vi "Actor Core.vi"(8 "error in":errorcluster, 11 "Panel Actor in":refnum<class "Panel Actor.lvclass">) -> (0 "error out":errorcluster, 3 "Actor out":refnum<class "Actor.lvclass">)   [LabVIEW 2023, in "Panel Actor.lvlib" / "Panel Actor.lvclass"]
doc: "The user interface for this panel.\n\n----\nPlease see the following web address for additional documentation and tutorial information:\nhttp://www.mooregoodideas.com/mgi-panel-manager/\n\nAuthor: Derek Trepanier\n\nCopyright (c) 2018, Moore Good Ideas, Inc.\n\nAll rights reserved.\n\nRedistribution and use in source and binary forms, with or without modification, are permitted provided that the following conditions are met:\n\n * Redistributions of source code must retain the above copyright notice, this list of conditions and the following disclaimer.\n * Redistributions in binary form must reproduce the above copyright notice, this list of conditions and the following disclaimer in the documentation and/or other materials provided with the distribution.\n * Neither the name of Moore Good Ideas, Inc. nor the names of its contributors may be used to endorse or promote products derived from this software without specific prior written permission.\n\nTHIS SOFTWARE IS PROVIDED BY THE COPYRIGHT HOLDERS AND CONTRIBUTORS \"AS IS\" AND ANY EXPRESS OR IMPLIED WARRANTIES, INCLUDING, BUT NOT LIMITED TO, THE IMPLIED WARRANTIES OF MERCHANTABILITY AND FITNESS FOR A PARTICULAR PURPOSE ARE DISCLAIMED. IN NO EVENT SHALL THE COPYRIGHT OWNER OR CONTRIBUTORS BE LIABLE FOR ANY DIRECT, INDIRECT, INCIDENTAL, SPECIAL, EXEMPLARY, OR CONSEQUENTIAL DAMAGES (INCLUDING, BUT NOT LIMITED TO, PROCUREMENT OF SUBSTITUTE GOODS OR SERVICES; LOSS OF USE, DATA, OR PROFITS; OR BUSINESS INTERRUPTION) HOWEVER CAUSED AND ON ANY THEORY OF LIABILITY, WHETHER IN CONTRACT, STRICT LIABILITY, OR TORT (INCLUDING NEGLIGENCE OR OTHERWISE) ARISING IN ANY WAY OUT OF THE USE OF THIS SOFTWARE, EVEN IF ADVISED OF THE POSSIBILITY OF SUCH DAMAGE."
uses:
  Library/Panel Actor.lvclass
  Panel/Panel/Panel.lvclass
  builds/Framework/Monitored Actor.lvlibp/Actor Monitor/Actor Monitor/Actor Monitor.lvclass
  builds/Framework/Actor Framework.lvlibp/1abvi3w/vi.lib/ActorFramework/Actor/Actor.lvclass
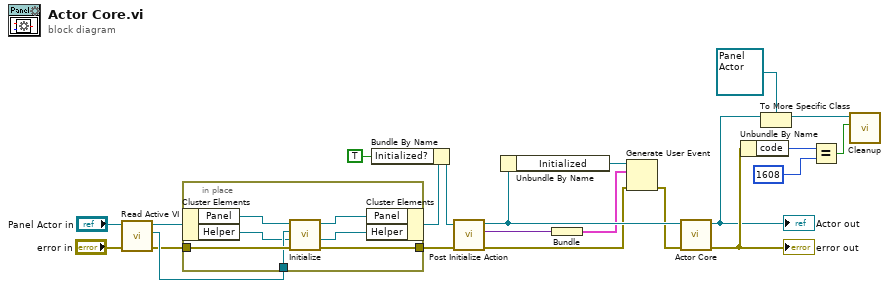
[diagram p0: block diagram]
diagram:
  n1 = call "Read Active VI.vi"("error in (no error)"="error in", "Panel Actor in"="Panel Actor in") -> ("error out"=w12:errorcluster, "Active VI ref"=w14:refnum<vi>, "Panel Actor out"=w15:refnum<class "Panel Actor.lvclass">)  [unwired: 7 in]
  n2 = in-place {
    in-place-border: w12 -> [w29]
    in-place-border: w14 -> [w27]
    in-place-border: [w26] -> w22
    n3 = in-place-cluster #1(w15) -> ("Panel"=w28:refnum<class "Panel.lvclass">, "Helper"=w23:refnum<class "Panel Helper.lvclass">)
    n4 = call "Initialize.vi"("error in (no error)"=w29, "My Helper in"=w23, "VI Refnum"=w27, "Panel In"=w28) -> ("error out"=w26:errorcluster, "My Helper out"=w24:refnum<class "Panel Helper.lvclass">, "Panel Out"=w25:refnum<class "Panel.lvclass">)  [unwired: 5 in]
    n5 = in-place-cluster #1("Panel"=w25, "Helper"=w24) -> (w20:refnum<class "Panel Actor.lvclass">)
  }
  n6 = Bundle By Name(cluster=w20, "Initialized?"=TRUE) -> (w8:refnum<class "Panel Actor.lvclass">)
  n7 = call-dynamic "Post Initialize Action.vi"("error in (no error)"=w22, "Panel Actor in"=w8) -> ("error out"=w4:errorcluster, "Init Event Data"=w2:variant, "Panel Actor out"=w6:refnum<class "Panel Actor.lvclass">)  [unwired: 7 in]
  n8 = Unbundle By Name(w6) -> ("Initialized"=w5:refnum<user-event>)
  n9 = Bundle("Init Event Data"=w2) -> (w1:cluster{"Init Event Data":variant})  [unwired: 1 in]
  n10 = Generate User Event(user event=w5, event data cluster=w1, error in=w4) -> (error out=w3:errorcluster)  [unwired: 1 in, 1 out]
  n11 = call-parent "Actor Core.vi"("error in"=w3, "Actor in"=w6) -> ("error out"=w19:errorcluster, "Actor out"=w10:refnum<class "Actor.lvclass">)  [unwired: 8 in]
  "error out" <- w19
  "Actor out" <- w10
  n12 = Unbundle By Name(w19) -> ("code"=w18:i32)
  n13 = To More Specific Class(target class=refnum<class "Panel Actor.lvclass"> refnum ("Panel Actor.lvlib:Panel Actor.lvclass"), reference=w10) -> (specific class reference=w9:refnum<class "Panel Actor.lvclass">)  [unwired: 1 in, 1 out]
  n14 = Equal?(x=w18, y=1608) -> (x = y?=w17:bool)
  n15 = call "Cleanup.vi"("Critical Stop?"=w17, "Panel Actor in"=w9) -> ()  [unwired: 10 in]
